vi "Read Fill Spacing.vi"(8 "error in (no error)":errorcluster, 11 "Rectangle Settings in":refnum<class "Rectangle Settings.lvclass">) -> (0 "error out":errorcluster, 2 "Fill Spacing":dbl, 3 "Rectangle Settings out":refnum<class "Rectangle Settings.lvclass">)   [LabVIEW 2019, in "Rectangle Settings.lvclass"]
uses:
  Rectangle Settings.lvclass
  Rectangle Settings.lvclass/Rectangle Settings.ctl
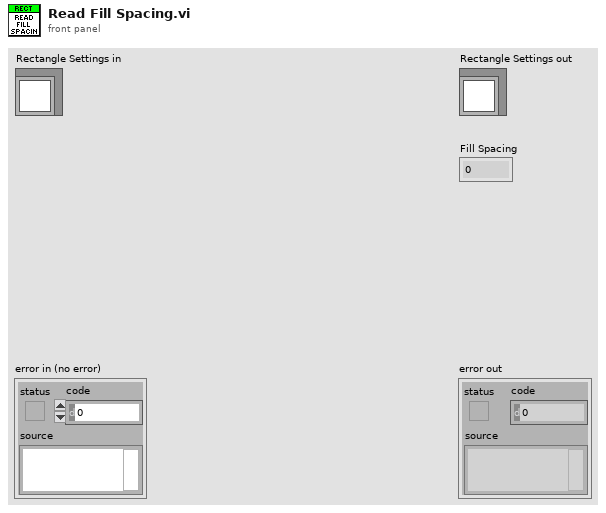
[diagram p1: front panel]
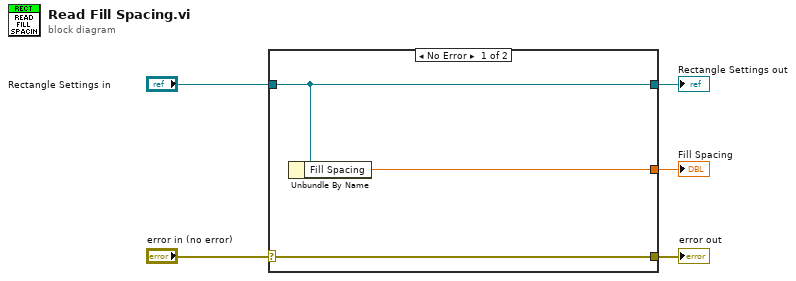
[diagram p0: block diagram]
diagram:
  n1 = case shown="No Error" "error in (no error)" {
    selector: "error in (no error)" -> [w8 w9]
    tunnel: [w8 w9] -> w4
    tunnel: [w7 w10] -> w2
    tunnel: "Rectangle Settings in" -> [w7 w10]
    tunnel: [w6 _] -> w1
    frame No Error {
      n2 = Unbundle By Name(w7) -> ("Fill Spacing"=w6:dbl)
    }
    frame Error {
    }
  }
  "error out" <- w4
  "Rectangle Settings out" <- w2
  "Fill Spacing" <- w1
